vi "change tag name.vi"(8 "error in":errorcluster, 9 "new name":string, 10 "old name":string, 11 "shared memory module configuration":refnum<class "shared memory configuration.lvclass">) -> (0 "error out":errorcluster, 1 "new channels":refnum<class "TBM channel.lvclass">[](array[class]), 2 "old channels":refnum<class "TBM channel.lvclass">[](array[class]), 3 "shared memory module configuration out":refnum<class "shared memory configuration.lvclass">)   [LabVIEW 2013, in "Shared Memory Configuration.lvclass"]
doc: "***TODO***\n\n<B>Input Parameters</B>\n\n<B>error in</B> describes error conditions that occur before this node runs. This input provides standard error in functionality.\n\n<B>new name</B> ***TODO***new name\n\n<B>old name</B> ***TODO***old name\n\n<B>shared memory module configuration</B> ***TODO***shared memory module configuration\n\n<B>Output Parameters</B>\n\n<B>error out</B> contains error information. This output provides standard error out functionality.\n\n<B>new channels</B> ***TODO***new channels\n\n<B>old channels</B> ***TODO***old channels\n\n<B>shared memory module configuration out</B> ***TODO***shared memory module configuration out"
uses:
  shared memory configuration.lvclass
  <vilib>/NI/Tag Bus Module Framework/channel/TBM channel.lvclass
  shared memory configuration.lvclass/shared memory configuration.ctl
  <vilib>/NI/Tag Bus/tag/tag descriptor.lvclass/tag descriptor.ctl
  <vilib>/NI/Tag Bus/tag/tag descriptor.lvclass
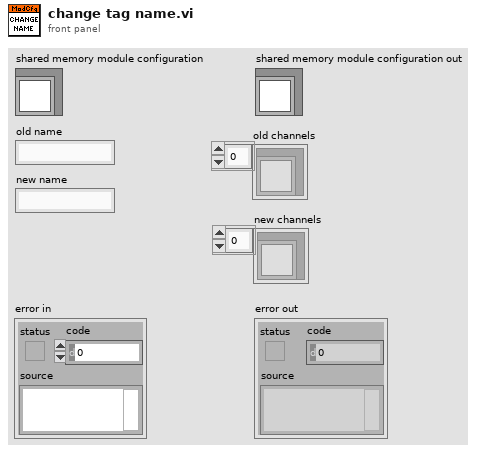
[diagram p1: front panel]
types:
  T1 = typedef "shared memory configuration.lvclass/Line.ctl" = cluster{"name":string, "data type":T2, "channel":refnum<class "TBM channel.lvclass">}
  T2 = typedef "tag bus.lvlib/tag descriptor.lvclass/Data Type.ctl" = enum16{"Double", "Single", "I64", "I32", "I16", "I8", "U64", "U32", "U16", "U8", "Boolean", "String", "Array of Double", "Array of Single", "Array of I64", "Array of I32", "Array of I16", "Array of I8", "Array of U64", "Array of U32", "Array of U16", "Array of U8", "Array of Boolean", "Array of String"}
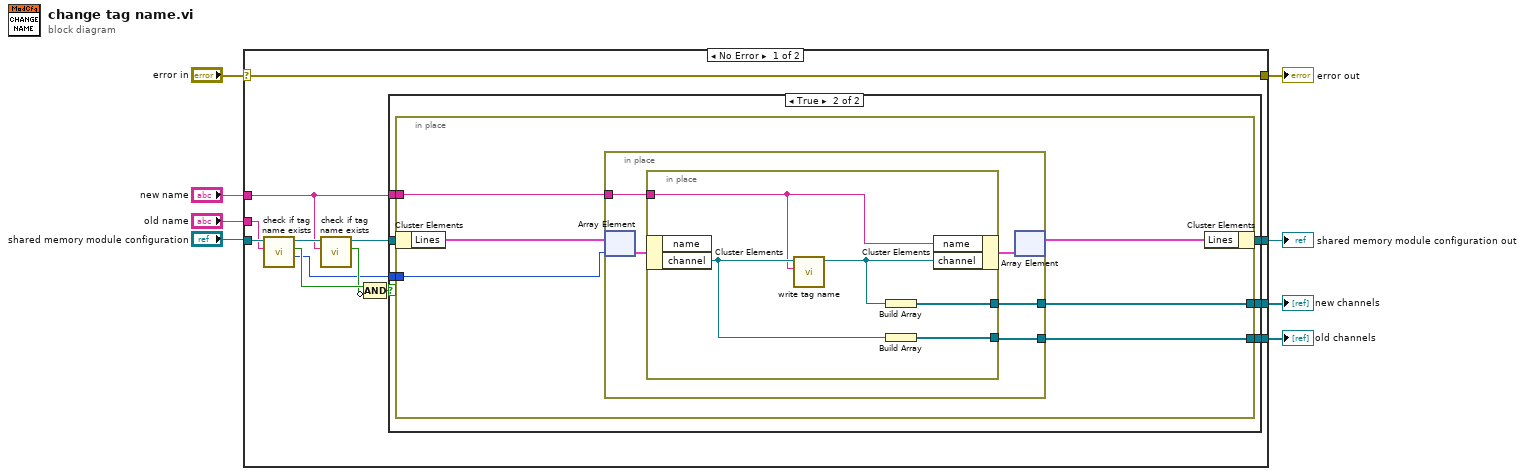
[diagram p0: block diagram]
diagram:
  n1 = case shown="No Error" "error in" {
    selector: "error in" -> [w21 w46]
    tunnel: [w21 w46] -> w7
    tunnel: [w18 w45] -> w6
    tunnel: "shared memory module configuration" -> [w20 w45]
    tunnel: "old name" -> [w19 _]
    tunnel: "new name" -> [w11 _]
    tunnel: [w10 _] -> w3
    tunnel: [w9 _] -> w2
    frame No Error {
      n2 = call "check if tag name exists.vi"("name to locate"=w19, "shared memory module configuration in"=w20) -> ("index"=w12:i32, "found?"=w15:bool, "shared memory module configuration out"=w17:refnum<class "shared memory configuration.lvclass">)  [unwired: 6 in, 1 out]
      n3 = call "check if tag name exists.vi"("name to locate"=w11, "shared memory module configuration in"=w17) -> ("found?"=w14:bool, "shared memory module configuration out"=w16:refnum<class "shared memory configuration.lvclass">)  [unwired: 6 in, 2 out]
      n4 = Compound Arithmetic op=AND(w15, invert w14) -> (w13:bool)
      n5 = case shown="True" w13 {
        tunnel: w16 -> [w22 w28]
        tunnel: [w22 w27] -> w18
        tunnel: w12 -> [_ w26]
        tunnel: w11 -> [_ w25]
        tunnel: [_ w24] -> w10
        tunnel: [_ w23] -> w9
        frame False {
        }
        frame True {
          n6 = in-place {
            in-place-border: w26 -> [w32]
            in-place-border: w25 -> [w31]
            in-place-border: [w30] -> w24
            in-place-border: [w29] -> w23
            n7 = in-place-cluster #1(w28) -> ("Lines"=w34:T1[])
            n8 = in-place {
              in-place-border: w31 -> [w38]
              in-place-border: [w36] -> w30
              in-place-border: [w35] -> w29
              n9 = in-place-array #2(w34, w32) -> (w39:T1)
              n10 = in-place {
                in-place-border: w38 -> [w41]
                in-place-border: [w43] -> w36
                in-place-border: [w44] -> w35
                n11 = in-place-cluster #3(w39) -> ("channel"=w42:refnum<class "TBM channel.lvclass">)  [unwired: 1 out]
                n12 = call <vilib>:"write tag name.vi"("name"=w41, "system tag in"=w42) -> ("system tag out"=w40:refnum<class "TBM channel.lvclass">)  [unwired: 8 in, 1 out]
                n13 = Build Array(w40) -> (w43:refnum<class "TBM channel.lvclass">[])
                n14 = Build Array(w42) -> (w44:refnum<class "TBM channel.lvclass">[])
                n15 = in-place-cluster #3("name"=w41, "channel"=w40) -> (w37:T1)
              }
              n16 = in-place-array #2(w37) -> (w33:T1[])  [unwired: 1 out]
            }
            n17 = in-place-cluster #1("Lines"=w33) -> (w27:refnum<class "shared memory configuration.lvclass">)
          }
        }
      }
    }
    frame Error {
    }
  }
  "error out" <- w7
  "shared memory module configuration out" <- w6
  "new channels" <- w3
  "old channels" <- w2
